vi "Replace Arguments.vi"(1 "Arguments":string[](array[string]), 2 "Message":string) -> (0 "Output Message":string)   [LabVIEW 2019, in "TSC Event Logger.lvlib" / "Layout.lvclass"]
uses:
  Layout.lvclass
  <vilib>/regexp/Match Regular Expression.xnode
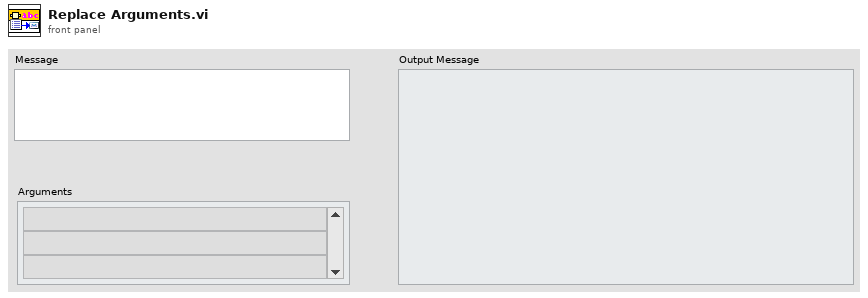
[diagram p1: front panel]
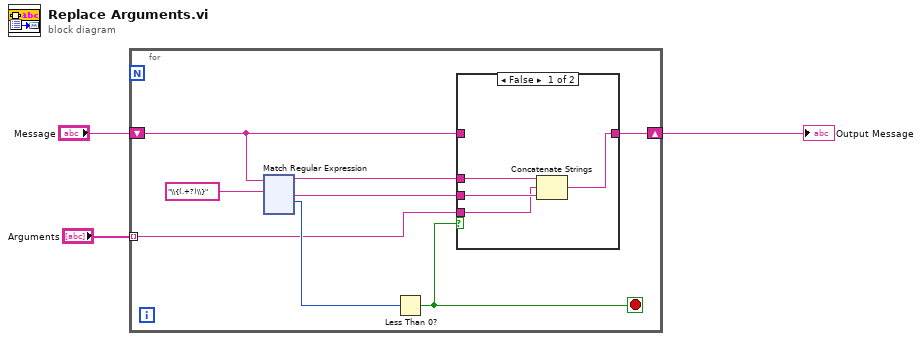
[diagram p0: block diagram]
diagram:
  n1 = for {
    tunnel: "Arguments" -> [w4] mode=indexing
    shift-right: [w7] -> w3
    shift-left: "Message" -> [w8]
    stop <- w9 stop-if-true
    n2 = xnode "Match Regular Expression"("input string"=w8, "regular expression"="\\{(.+?)\\}") -> ("before match"=w6:string, "after match"=w5:string, "offset past match"=w10:i32)  [unwired: 4 in, 2 out]
    n3 = Less Than 0?(x=w10) -> (x < 0?=w9:bool)
    n4 = case shown="False" w9 {
      tunnel: w8 -> [_ w16]
      tunnel: [w12 w16] -> w7
      tunnel: w6 -> [w15 _]
      tunnel: w5 -> [w14 _]
      tunnel: w4 -> [w13 _]
      frame False {
        n5 = Concatenate Strings(w15, w13, w14) -> (w12:string)
      }
      frame True {
      }
    }
  }
  "Output Message" <- w3
